vi "PH_Sixpack_Switch.destructor.vi"(0 "i ref in":refnum<vi>, 5 "error in(no error)":errorcluster) -> (19 "error out":errorcluster)   [LabVIEW 2014, in "PH_Sixpack_Switch.lvlib"]
doc: "This is the destructor of a class.\n\nLicense Agreement for this software:\n\nCopyright (C)\nGesellschaft für Schwerionenforschung, GSI\nPlanckstr. 1\n64291 Darmstadt\nGermany\n\nContact: D.Beck@gsi.de \n\nThis program is free software; you can redistribute it and/or modify it under the terms of the \nGNU General Public License as published by the Free Software Foundation; either version 2 of \nthe license, or (at your option) any later version.\n\nThis program is distributed in the hope that it will be useful, but WITHOUT ANY WARRANTY; \nwithout even the implied warranty of MERCHANTABILITY or FITNESS FOR A PARTICULAR PURPOSE. See the GNU General License for more details (http://www.gnu.org).\n\nGesellschaft für Schwerionenforschung, GSI\nPlanckstr. 1, 64291 Darmstadt, Germany\nFor all questions and ideas contact: M.Richter@gsi.de, H.Brand@gsi.de or D.Beck@gsi.de.\nLast update: 16-JUN-2004"
uses:
  PH_Sixpack_Switch.lvlib
  PH_Basics/PH_AxisGUI_BaseClass/PH_AxisGUI_BaseClass.lvlib
  PH_Basics/PH_PSDBWriter/PH_PSDBWriter.lvlib
  PH_Basics/PH_StatusHandler/PH_StatusHandler.lvlib
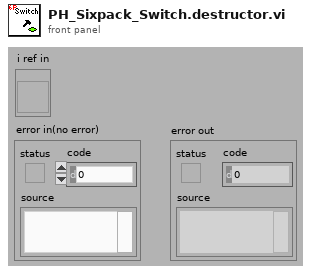
[diagram p1: front panel]
types:
  T1 = enum16{"SetAttribute", "GetAttribute", "CreateAttribute", "DestroyAttribute", "DestroyAllAtributes"}
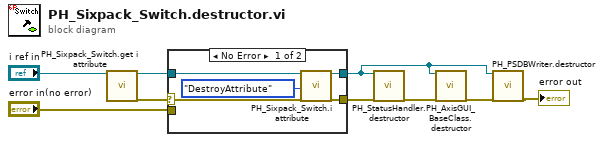
[diagram p0: block diagram]
diagram:
  n1 = call "PH_Sixpack_Switch.get i attribute.vi"("i ref in"="i ref in") -> ("i ref out"=w8:refnum<vi>, "error out"=w7:errorcluster)  [unwired: 16 in, 1 out]
  n2 = case shown="No Error" w7 {
    selector: w7 -> [w10 _]
    tunnel: [w13 w16] -> w5
    tunnel: w8 -> [w12 w15]
    tunnel: [w11 w15] -> w1
    tunnel: "error in(no error)" -> [_ w16]
    frame No Error {
      n3 = call "PH_Sixpack_Switch.i attribute.vi"("VI Refnum"=w12, "Action"=T1."DestroyAttribute", "error in (no error)"=w10) -> ("VI Refnum out"=w11:refnum<vi>, "error out"=w13:errorcluster)  [unwired: 14 in, 1 out]
    }
    frame Error {
    }
  }
  n4 = call "PH_StatusHandler.destructor.vi"("i ref in"=w1, "error in(no error)"=w5) -> ("error out"=w2:errorcluster)  [unwired: 17 in]
  n5 = call "PH_AxisGUI_BaseClass.destructor.vi"("i ref in"=w1, "error in(no error)"=w2) -> ("error out"=w4:errorcluster)  [unwired: 17 in]
  n6 = call "PH_PSDBWriter.destructor.vi"("i ref in"=w1, "error in(no error)"=w4) -> ("error out"=→"error out":errorcluster)  [unwired: 17 in]
